vi "Send Message - Add Error.vi"(7 "Source":string, 8 "error in (no error)":errorcluster, 11 "Error to Handle":errorcluster) -> (0 "error out":errorcluster)   [LabVIEW 2010, in "Error Handler.lvlib"]
doc: "Sends a Stop message to the Module loop"
uses:
  Error Handler.lvlib
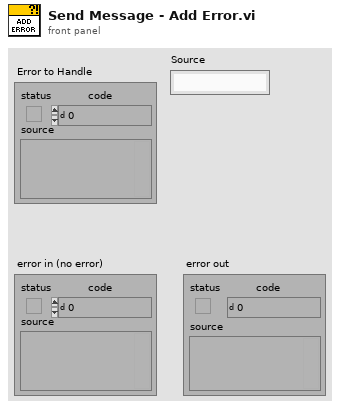
[diagram p1: front panel]
types:
  T1 = cluster{"Source":string, "Error to Handle":errorcluster}
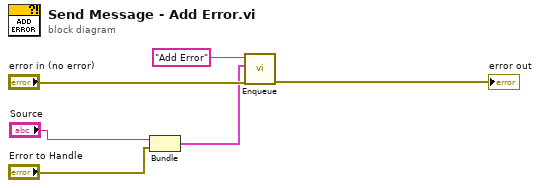
[diagram p0: block diagram]
diagram:
  n1 = Bundle("Source"="Source", "Error to Handle"="Error to Handle") -> (w1:T1)  [unwired: 1 in]
  n2 = call "Enqueue.vi"("error in (no error)"="error in (no error)", "Data"=w1, "Message"="Add Error") -> ("error out"=→"error out":errorcluster)  [unwired: 8 in]
